vi "Set Washer Status.vi"(10 "Dryer":T1 {"Day Cycle Count" format="%04d"}, 11 "Debug Log":string) -> (3 "Dryer 2":T1 {"Day Cycle Count" format="%04d"})   [LabVIEW 2012]
uses:
  Washer.ctl
  Washer Details.ctl
  Washer Status Ctrl.ctl
  Globals HCC.vi
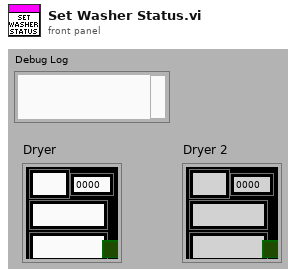
[diagram p1: front panel]
types:
  T1 = typedef "Washer.ctl" = cluster{"Serial Number":string, "Day Cycle Count":i32, "Station Label":string, "Sample Record(t, CC, Tc, ASCII, Status, L1,L2,Trmb,V{,V2,SW} ) ":string[], "Hist Record(Cycle Count, t-comp,L1max, L2max, Tmax) ":string[][], "Status Color":u32, "Current Run Start Time":dbl, "Station Index":i32, "Audit Alert":bool, "Washer Details":T2, "Board ID":string, "Boolean":bool, "Status":T3}
  T2 = typedef "Washer Details.ctl" = cluster{"Cycle Count":string, "Status":string, "Debug ASCII":string, "Notes":string, "Lab ID":string, "Total Time On":string, "TR Number":string}
  T3 = typedef "Washer Status Ctrl.ctl" = enum16{"Cycle Not Started", "Cycle Running", "Paused", "Cycle Completed", "Eval Mode Entered", "Err"}
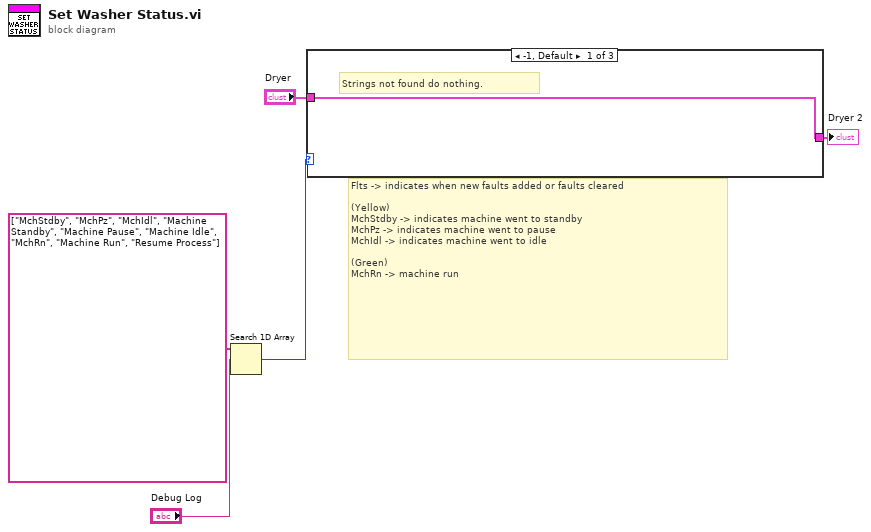
[diagram p0: block diagram]
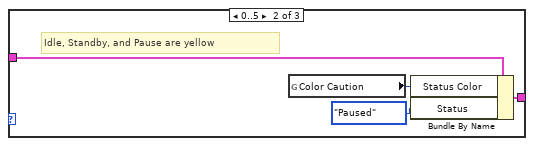
[diagram p2: hidden frame]
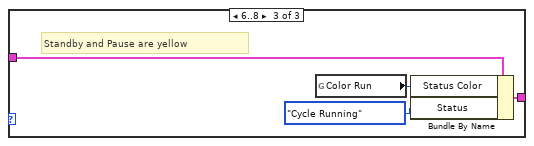
[diagram p3: hidden frame]
diagram:
  # "Flts -> indicates when new faults added or faults cleared\n\n(Yellow)\nMchStdby -> indicates machine went to standby\nMchPz -> indicates machine went to pause\nMchIdl -> indicates machine went to idle \n\n(Green)\nMchRn -> machine run"
  n1 = Search 1D Array(1D array=string[] ["MchStdby", "MchPz", "MchIdl", "Machine Standby", "Machine Pause", "Machine Idle", "MchRn", "Machine Run", "Resume Process"] ("operators (none)"), element="Debug Log") -> (index of element=w1:i32)  [unwired: 1 in]
  n2 = case shown="-1, Default" w1 {
    tunnel: [w6 w8 w12] -> w4
    tunnel: "Dryer" -> [w6 w10 w14]
    frame -1, Default {
      # "Strings not found do nothing."
    }
    frame 0..5 {
      # "Idle, Standby, and Pause are yellow"
      n3 = global read "Globals HCC.vi" "Color Caution"() -> (w9:u32)
      n4 = Bundle By Name(cluster=w10, "Status Color"=w9, "Status"=Washer_Status_Ctrl."Paused") -> (w8:T1)
    }
    frame 6..8 {
      # "Standby and Pause are yellow"
      n5 = global read "Globals HCC.vi" "Color Run"() -> (w13:u32)
      n6 = Bundle By Name(cluster=w14, "Status Color"=w13, "Status"=Washer_Status_Ctrl."Cycle Running") -> (w12:T1)
    }
  }
  "Dryer 2" <- w4
